vi "Rhino Test.vi"(8 "Test Progress":dbl, 9 "Test Progress Text":string) -> ()   [LabVIEW 2018]
uses:
  Climb/Implementation/Climb Operations.ctl
  <vilib>/Rock Robotics/Network Tables/NT Write String.vi
  <vilib>/Rock Robotics/WPI/ThirdParty/Phoenix-LabVIEW/Motor Controller/Get/CTRE_Phoenix_MotorController_GetSelectedSensorData.vi
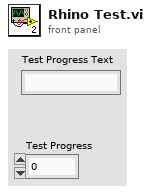
[diagram p1: front panel]
types:
  T1 = typedef "Climb Operations.ctl" = enum16{"Reserve", "Read Current", "Immediate", "Ready", "Auto-Climb", "Reset/Turbo-Tilt", "Manual Climb"}
  T2 = typedef "Command Status Info.ctl" = cluster{"Name":string, "Status":T3, "notifier out":T4}
  T3 = typedef "Completion Status.ctl" = enum16{"Successful", "Aborted", "Incomplete"}
  T4 = typedef "Completion Notifier.ctl" = refnum<notifier>
  T5 = typedef "WPI_MotorControlDeviceRef.ctl" = cluster{"DeviceStatus":errorcluster, "Type":T6, "PWM":cluster{"PWM Channel":T7, "DeadBand":T8}, "CAN":cluster{"Device Number":u8, "SetOutput VI Ref":variant, "GetOutput VI Ref":variant, "Enable VI Ref":variant, "Disable VI Ref":variant, "Data":variant}, "Invert":bool, "DIO PWM":cluster{"PWM \"Enable\" Channel":T7, "DIOChannel":T9, "PWM Rate":dbl}}
  T6 = typedef "WPI_MotorControlType.ctl" = enum16{"PWM", "CAN", "DIO PWM"}
  T7 = typedef "FPGA_DIOPWMChannel.ctl" = enum8{"PWM 0", "PWM 1", "PWM 2", "PWM 3", "PWM 4", "PWM 5", "PWM 6", "PWM 7", "PWM 8", "PWM 9", "PWM MXP 0", "PWM MXP 1", "PWM MXP 2", "PWM MXP 3", "PWM MXP 4", "PWM MXP 5", "PWM MXP 6", "PWM MXP 7", "PWM MXP 8", "PWM MXP 9", "Invalid"}
  T8 = typedef "WPI_PWMDeadband.ctl" = cluster{"Name":string, "maxPositivePwm":i32, "minPositivePwm":i32, "centerPwm":i32, "maxNegativePwm":i32, "minNegativePwm":i32, "angularRange":u16}
  T9 = typedef "FPGA_DIOChannel.ctl" = enum8{"DIO 0", "DIO 1", "DIO 2", "DIO 3", "DIO 4", "DIO 5", "DIO 6", "DIO 7", "DIO 8", "DIO 9", "DIO MXP 0", "DIO MXP 1", "DIO MXP 2", "DIO MXP 3", "DIO MXP 4", "DIO MXP 5", "DIO MXP 6", "DIO MXP 7", "DIO MXP 8", "DIO MXP 9", "DIO MXP 10", "DIO MXP 11", "DIO MXP 12", "DIO MXP 13", "DIO MXP 14", "DIO MXP 15", "SPI Port CS1", "SPI Port CS2", "SPI Port CS3", "SPI Port MISO", "SPI Port MOSI", "Invalid"}
  T10 = typedef "WPI_SwitchDevRef.ctl" = cluster{"DevStatus":errorcluster, "DIO Channel":T9, "CntIndex":T11, "Normally Closed":bool}
  T11 = typedef "FPGA_CounterCtrSystemIndex.ctl" = enum8{"Ctr 0", "Ctr 1", "Ctr 2", "Ctr 3", "Ctr 4", "Ctr 5", "Ctr 6", "Ctr 7", "Invalid"}
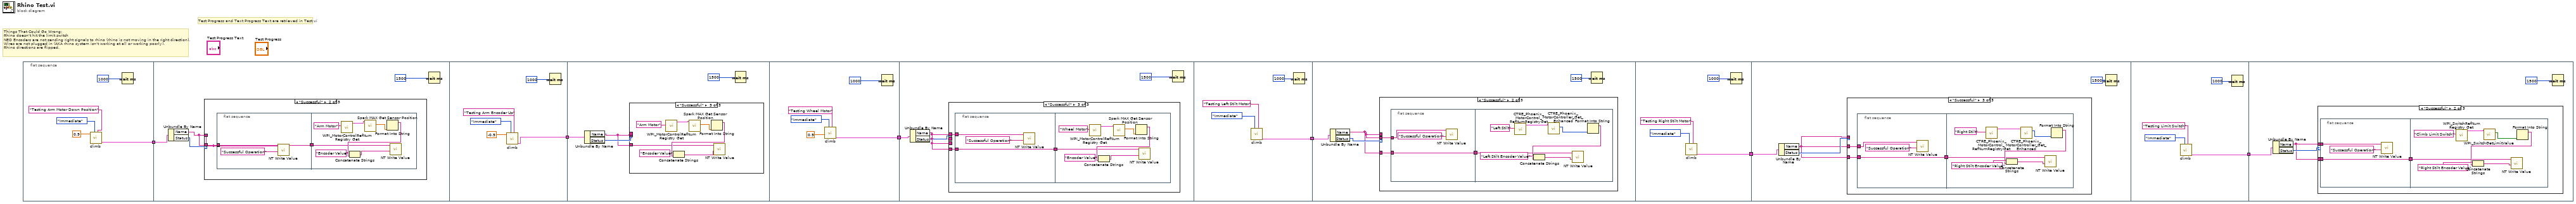
[diagram p0: block diagram]
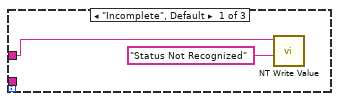
[diagram p2: hidden frame]
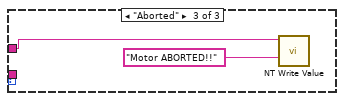
[diagram p3: hidden frame]
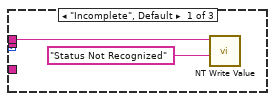
[diagram p4: hidden frame]
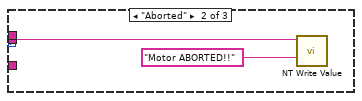
[diagram p5: hidden frame]
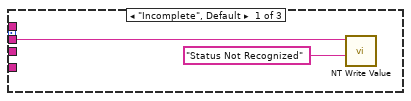
[diagram p6: hidden frame]
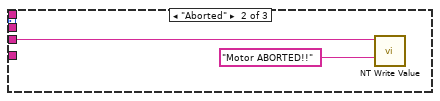
[diagram p7: hidden frame]
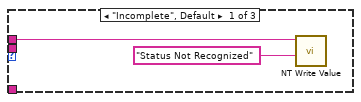
[diagram p8: hidden frame]
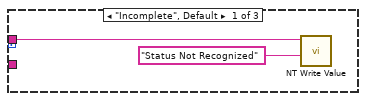
[diagram p10: hidden frame]
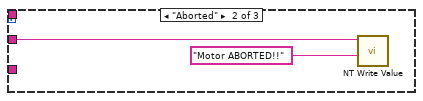
[diagram p11: hidden frame]
diagram:
  # "Test Progress and Text Progress Text are retrieved in Test.vi"
  # "Things That Could Go Wrong:\nRhino doesn't hit the limit switch\nNEO Encoders are not sending right signals to rhino (rhino is not moving in the right direction).\nWires are not plugged in (AKA rhino system isn't working at all or working poorly).\nRhino directions are flipped."
  n1 = flat-sequence {
    tunnel: [w9] -> w6
    tunnel: w6 -> [w12]
    tunnel: [w36] -> w5
    tunnel: w5 -> [w38]
    tunnel: [w53] -> w4
    tunnel: w4 -> [w58]
    tunnel: [w79] -> w3
    tunnel: w3 -> [w83]
    tunnel: [w102] -> w2
    tunnel: w2 -> [w106]
    tunnel: [w129] -> w1
    tunnel: w1 -> [w131]
    frame #0 {
      n2 = call "climb.vi"("Description"="Testing Arm Motor Down Position", "Operation"=Climb_Operations."Immediate", "Setpoint ARM"=0.9) -> ("Command Info Out"=w9:T2)  [unwired: 8 in]
      n3 = Wait (ms)(milliseconds to wait=u32 1000) -> ()  [unwired: 1 out]
    }
    frame #1 {
      n4 = Unbundle By Name(w12) -> ("Name"=w13:string, "Status"=w14:T3)
      n5 = case shown="\"Successful\"" w14 {
        tunnel: w13 -> [w17 w20 w32]
        tunnel: w13 -> [_ w19 _]
        frame "Incomplete", Default {
          n6 = call-poly <vilib>:"NT Write Value.vi"("String"="Status Not Recognized", "Name"=w17) -> ()  [unwired: 9 in, 1 out]
        }
        frame "Successful" {
          n7 = flat-sequence {
            tunnel: w20 -> [w22]
            tunnel: w20 -> [_]
            tunnel: w19 -> [w21]
            tunnel: [w21] -> w18
            tunnel: w18 -> [w26]
            frame #0 {
              n8 = call-poly <vilib>:"NT Write Value.vi"("String"="Successful Operation", "Name"=w22) -> ()  [unwired: 9 in, 1 out]
            }
            frame #1 {
              n9 = call <vilib>:"WPI_MotorControlRefNum Registry Get.vi"("refnum name"="Arm Motor") -> ("MotorControlDevRef"=w24:T5)  [unwired: 9 in, 1 out]
              n10 = call <vilib>:"Spark MAX Get Sensor Position.vi"("MotorControlDevRef in"=w24) -> ("Sensor Position"=w30:dbl)  [unwired: 7 in, 3 out]
              n11 = Format Into String(w30) -> (resulting string=w29:string)  [unwired: 3 in, 1 out]
              n12 = Concatenate Strings("Encoder Value" ("string"), w29) -> (w27:string)
              n13 = call-poly <vilib>:"NT Write Value.vi"("String"=w27, "Name"=w26) -> ()  [unwired: 9 in, 1 out]
            }
          }
        }
        frame "Aborted" {
          n14 = call-poly <vilib>:"NT Write Value.vi"("String"="Motor ABORTED!!", "Name"=w32) -> ()  [unwired: 9 in, 1 out]
        }
      }
      n15 = Wait (ms)(milliseconds to wait=u32 1500) -> ()  [unwired: 1 out]
    }
    frame #2 {
      n16 = call "climb.vi"("Description"="Testing Arm Encoder Up", "Operation"=Climb_Operations."Immediate", "Setpoint ARM"=-0.9) -> ("Command Info Out"=w36:T2)  [unwired: 8 in]
      n17 = Wait (ms)(milliseconds to wait=u32 1000) -> ()  [unwired: 1 out]
    }
    frame #3 {
      n18 = Unbundle By Name(w38) -> ("Name"=w39:string, "Status"=w40:T3)
      n19 = case shown="\"Successful\"" w40 {
        tunnel: w39 -> [_ w44 _]
        tunnel: w39 -> [w43 _ _]
        tunnel: w39 -> [_ _ w48]
        frame "Incomplete", Default {
          n20 = call-poly <vilib>:"NT Write Value.vi"("String"="Status Not Recognized", "Name"=w43) -> ()  [unwired: 9 in, 1 out]
        }
        frame "Aborted" {
          n21 = call-poly <vilib>:"NT Write Value.vi"("String"="Motor ABORTED!!", "Name"=w44) -> ()  [unwired: 9 in, 1 out]
        }
        frame "Successful" {
          n22 = call <vilib>:"WPI_MotorControlRefNum Registry Get.vi"("refnum name"="Arm Motor") -> ("MotorControlDevRef"=w46:T5)  [unwired: 9 in, 1 out]
          n23 = call <vilib>:"Spark MAX Get Sensor Position.vi"("MotorControlDevRef in"=w46) -> ("Sensor Position"=w51:dbl)  [unwired: 7 in, 3 out]
          n24 = Format Into String(w51) -> (resulting string=w52:string)  [unwired: 3 in, 1 out]
          n25 = Concatenate Strings("Encoder Value" ("string"), w52) -> (w49:string)
          n26 = call-poly <vilib>:"NT Write Value.vi"("String"=w49, "Name"=w48) -> ()  [unwired: 9 in, 1 out]
        }
      }
      n27 = Wait (ms)(milliseconds to wait=u32 1500) -> ()  [unwired: 1 out]
    }
    frame #4 {
      n28 = call "climb.vi"("Description"="Testing Wheel Motor", "Operation"=Climb_Operations."Immediate", "Setpoint WHEELS"=0.9) -> ("Command Info Out"=w53:T2)  [unwired: 8 in]
      n29 = Wait (ms)(milliseconds to wait=u32 1000) -> ()  [unwired: 1 out]
    }
    frame #5 {
      n30 = Unbundle By Name(w58) -> ("Name"=w59:string, "Status"=w60:T3)
      n31 = case shown="\"Successful\"" w60 {
        tunnel: w59 -> [_ _ w68]
        tunnel: w59 -> [_ _ w67]
        tunnel: w59 -> [w62 _ _]
        tunnel: w59 -> [_ w64 _]
        frame "Incomplete", Default {
          n32 = call-poly <vilib>:"NT Write Value.vi"("String"="Status Not Recognized", "Name"=w62) -> ()  [unwired: 9 in, 1 out]
        }
        frame "Aborted" {
          n33 = call-poly <vilib>:"NT Write Value.vi"("String"="Motor ABORTED!!", "Name"=w64) -> ()  [unwired: 9 in, 1 out]
        }
        frame "Successful" {
          n34 = flat-sequence {
            tunnel: w68 -> [w70]
            tunnel: w67 -> [w69]
            tunnel: [w69] -> w66
            tunnel: w66 -> [w74]
            frame #0 {
              n35 = call-poly <vilib>:"NT Write Value.vi"("String"="Successful Operation", "Name"=w70) -> ()  [unwired: 9 in, 1 out]
            }
            frame #1 {
              n36 = call <vilib>:"WPI_MotorControlRefNum Registry Get.vi"("refnum name"="Wheel Motor") -> ("MotorControlDevRef"=w72:T5)  [unwired: 9 in, 1 out]
              n37 = call <vilib>:"Spark MAX Get Sensor Position.vi"("MotorControlDevRef in"=w72) -> ("Sensor Position"=w78:dbl)  [unwired: 7 in, 3 out]
              n38 = Format Into String(w78) -> (resulting string=w77:string)  [unwired: 3 in, 1 out]
              n39 = Concatenate Strings("Encoder Value" ("string"), w77) -> (w75:string)
              n40 = call-poly <vilib>:"NT Write Value.vi"("String"=w75, "Name"=w74) -> ()  [unwired: 9 in, 1 out]
            }
          }
        }
      }
      n41 = Wait (ms)(milliseconds to wait=u32 1500) -> ()  [unwired: 1 out]
    }
    frame #6 {
      n42 = call "climb.vi"("Description"="Testing Left Stilt Motor", "Operation"=Climb_Operations."Immediate") -> ("Command Info Out"=w79:T2)  [unwired: 9 in]
      n43 = Wait (ms)(milliseconds to wait=u32 1000) -> ()  [unwired: 1 out]
    }
    frame #7 {
      n44 = Unbundle By Name(w83) -> ("Name"=w84:string, "Status"=w86:T3)
      n45 = case shown="\"Successful\"" w86 {
        tunnel: w84 -> [_ w91 _]
        tunnel: w84 -> [_ w90 _]
        tunnel: w84 -> [w87 _ _]
        frame "Incomplete", Default {
          n46 = call-poly <vilib>:"NT Write Value.vi"("String"="Status Not Recognized", "Name"=w87) -> ()  [unwired: 9 in, 1 out]
        }
        frame "Successful" {
          n47 = flat-sequence {
            tunnel: w91 -> [w94]
            tunnel: w90 -> [w92]
            tunnel: [w92] -> w89
            tunnel: w89 -> [w97]
            frame #0 {
              n48 = call-poly <vilib>:"NT Write Value.vi"("String"="Successful Operation", "Name"=w94) -> ()  [unwired: 9 in, 1 out]
            }
            frame #1 {
              n49 = call <vilib>:"CTRE_Phoenix_MotorControl_RefNumRegistryGet.vi"("refnum name"="Left Stilt") -> ("PhoenixMotorControlDevRef"=w95:T5)  [unwired: 9 in, 1 out]
              n50 = call-poly <vilib>:"CTRE_Phoenix_MotorController_Get_Enhanced.vi"("PhoenixMotorControlDevRef"=w95) -> ("Position (Raw Sensor Units)"=w101:i32)  [unwired: 11 in, 3 out]
              n51 = Format Into String(w101) -> (resulting string=w99:string)  [unwired: 3 in, 1 out]
              n52 = Concatenate Strings("Left Stilt Encoder Value" ("string"), w99) -> (w98:string)
              n53 = call-poly <vilib>:"NT Write Value.vi"("String"=w98, "Name"=w97) -> ()  [unwired: 9 in, 1 out]
            }
          }
        }
        frame "Aborted" {
        }
      }
      n54 = Wait (ms)(milliseconds to wait=u32 1500) -> ()  [unwired: 1 out]
    }
    frame #8 {
      n55 = call "climb.vi"("Description"="Testing Right Stilt Motor", "Operation"=Climb_Operations."Immediate") -> ("Command Info Out"=w102:T2)  [unwired: 9 in]
      n56 = Wait (ms)(milliseconds to wait=u32 1000) -> ()  [unwired: 1 out]
    }
    frame #9 {
      n57 = Unbundle By Name(w106) -> ("Name"=w108:string, "Status"=w109:T3)
      n58 = case shown="\"Successful\"" w109 {
        tunnel: w108 -> [_ _ w115]
        tunnel: w108 -> [w110 _ _]
        tunnel: w108 -> [_ w112 w116]
        frame "Incomplete", Default {
          n59 = call-poly <vilib>:"NT Write Value.vi"("String"="Status Not Recognized", "Name"=w110) -> ()  [unwired: 9 in, 1 out]
        }
        frame "Aborted" {
          n60 = call-poly <vilib>:"NT Write Value.vi"("String"="Motor ABORTED!!", "Name"=w112) -> ()  [unwired: 9 in, 1 out]
        }
        frame "Successful" {
          n61 = flat-sequence {
            tunnel: w116 -> [w119]
            tunnel: w115 -> [w117]
            tunnel: [w117] -> w114
            tunnel: w114 -> [w122]
            frame #0 {
              n62 = call-poly <vilib>:"NT Write Value.vi"("String"="Successful Operation", "Name"=w119) -> ()  [unwired: 9 in, 1 out]
            }
            frame #1 {
              n63 = call <vilib>:"CTRE_Phoenix_MotorControl_RefNumRegistryGet.vi"("refnum name"="Right Stilt") -> ("PhoenixMotorControlDevRef"=w120:T5)  [unwired: 9 in, 1 out]
              n64 = call-poly <vilib>:"CTRE_Phoenix_MotorController_Get_Enhanced.vi"("PhoenixMotorControlDevRef"=w120) -> ("Position (Raw Sensor Units)"=w126:i32)  [unwired: 11 in, 3 out]
              n65 = Format Into String(w126) -> (resulting string=w124:string)  [unwired: 3 in, 1 out]
              n66 = Concatenate Strings("Right Stilt Encoder Value" ("string"), w124) -> (w123:string)
              n67 = call-poly <vilib>:"NT Write Value.vi"("String"=w123, "Name"=w122) -> ()  [unwired: 9 in, 1 out]
            }
          }
        }
      }
      n68 = Wait (ms)(milliseconds to wait=u32 1500) -> ()  [unwired: 1 out]
    }
    frame #10 {
      n69 = call "climb.vi"("Description"="Testing Limit Switch", "Operation"=Climb_Operations."Immediate") -> ("Command Info Out"=w129:T2)  [unwired: 9 in]
      n70 = Wait (ms)(milliseconds to wait=u32 1000) -> ()  [unwired: 1 out]
    }
    frame #11 {
      n71 = Unbundle By Name(w131) -> ("Name"=w132:string, "Status"=w133:T3)
      n72 = case shown="\"Successful\"" w133 {
        tunnel: w132 -> [_ w137 _]
        tunnel: w132 -> [_ w136 _]
        frame "Incomplete", Default {
        }
        frame "Successful" {
          n73 = flat-sequence {
            tunnel: w137 -> [w139]
            tunnel: w136 -> [w138]
            tunnel: [w138] -> w135
            tunnel: w135 -> [w143]
            frame #0 {
              n74 = call-poly <vilib>:"NT Write Value.vi"("String"="Successful Operation", "Name"=w139) -> ()  [unwired: 9 in, 1 out]
            }
            frame #1 {
              n75 = call <vilib>:"WPI_SwitchRefNum Registry Get.vi"("refnum name"="Climb Limit Switch") -> ("SwitchDevRef"=w141:T10)  [unwired: 9 in, 1 out]
              n76 = call <vilib>:"WPI_SwitchGetLimitValue.vi"("SwitchDevRef"=w141) -> ("Switch Pressed"=w145:bool)  [unwired: 8 in, 2 out]
              n77 = Format Into String(w145) -> (resulting string=w144:string)  [unwired: 3 in, 1 out]
              n78 = Concatenate Strings("Right Stilt Encoder Value" ("string"), w144) -> (w147:string)
              n79 = call-poly <vilib>:"NT Write Value.vi"("String"=w147, "Name"=w143) -> ()  [unwired: 9 in, 1 out]
            }
          }
        }
        frame "Aborted" {
        }
      }
      n80 = Wait (ms)(milliseconds to wait=u32 1500) -> ()  [unwired: 1 out]
    }
  }
